vi "Excel_Open.vi"(8 "error in (no error)":errorcluster, 10 "template (empty)":path, 11 "excel application":refnum<k7>) -> (0 "error out":errorcluster, 3 "references":T1)   [LabVIEW 2015]
doc: "自己改的打开报表的工具"
panel:
  in  "Excel._Worksheet":refnum<k7>
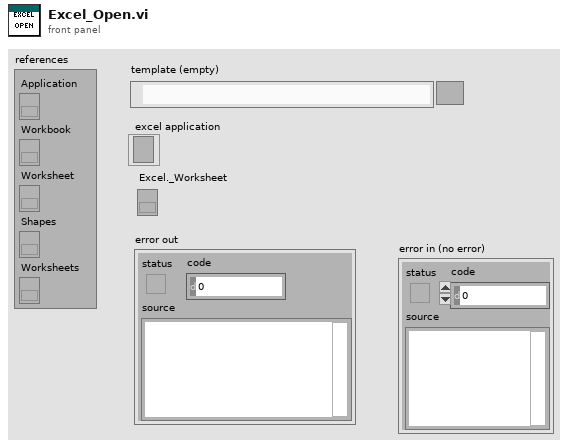
[diagram p1: front panel]
types:
  T1 = cluster{"Application":refnum<k7>, "Workbook":refnum<k7>, "Worksheet":refnum<k7>, "Shapes":refnum<k7>, "Worksheets":refnum<k7>}
  T2 = cluster{"excel application":refnum<k7>, "Add":refnum<k7>, "Excel._Worksheet":refnum<k7>, "Shapes":refnum<k7>, "Worksheets":refnum<k7>}
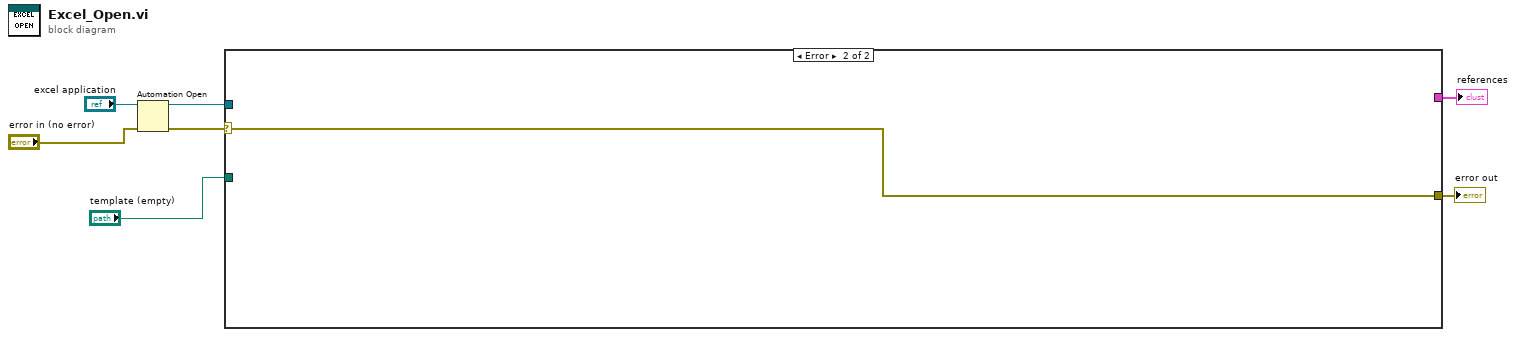
[diagram p0: block diagram]
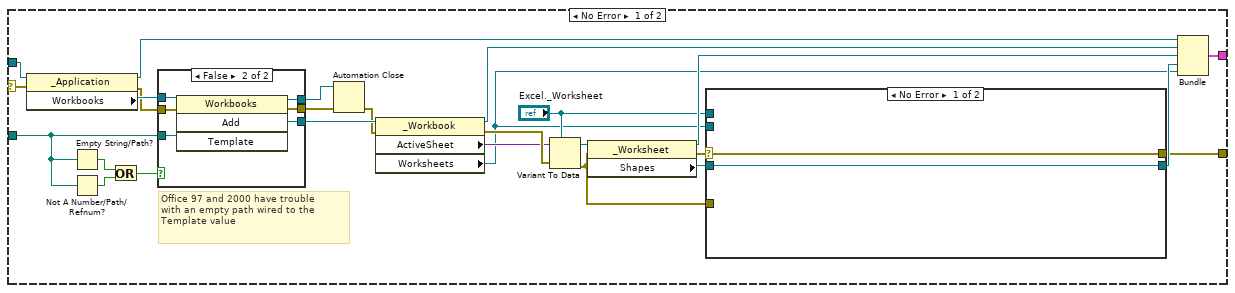
[diagram p2: hidden frame]
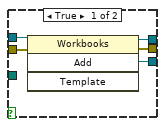
[diagram p3: hidden frame]
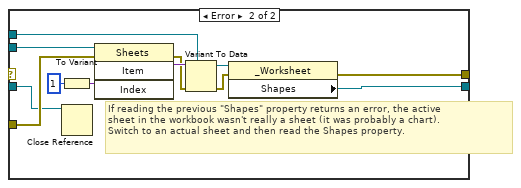
[diagram p4: hidden frame]
diagram:
  n1 = Automation Open(error in (no error)="error in (no error)", Automation Refnum="excel application") -> (Automation Refnum=w2:refnum<k7>, error out=w4:errorcluster)  [unwired: 2 in]
  n2 = case shown="Error" w4 {
    selector: w4 -> [w13 w59]
    tunnel: "template (empty)" -> [w12 _]
    tunnel: [w21 _] -> w6
    tunnel: [w16 w59] -> w3
    tunnel: w2 -> [w8 _]
    frame No Error {
      # "Office 97 and 2000 have trouble\nwith an empty path wired to the\nTemplate value"
      n3 = property class="_Application"(reference=w8, error in=w13) -> (reference out=w30:refnum<k7>, error out=w31:errorcluster, "Workbooks"=w32:refnum<k7>)
      n4 = Empty String/Path?(string/path=w12) -> (empty?=w11:bool)
      n5 = Not A Number/Path/Refnum?(number/path/refnum=w12) -> (NaN/Path/Refnum?=w10:bool)
      n6 = Or(x=w11, y=w10) -> (x .or. y?=w9:bool)
      n7 = case shown="False" w9 {
        tunnel: [w38 w44] -> w33
        tunnel: w32 -> [w37 w43]
        tunnel: w31 -> [w36 w42]
        tunnel: [w35 w41] -> w29
        tunnel: [w34 w40] -> w28
        tunnel: w12 -> [_ w39]
        frame True {
          n8 = invoke class="Workbooks" method="Add"(reference=w37, error in=w36) -> (reference out=w34:refnum<k7>, error out=w35:errorcluster, "Add"=w38:refnum<k7>)  [unwired: 2 in, 1 out]
        }
        frame False {
          n9 = invoke class="Workbooks" method="Add"(reference=w43, error in=w42, "Template"=w39) -> (reference out=w40:refnum<k7>, error out=w41:errorcluster, "Add"=w44:refnum<k7>)  [unwired: 1 in, 1 out]
        }
      }
      n10 = Automation Close(3:w29, 5:w28) -> (0:w27:errorcluster)
      n11 = property class="_Workbook"(reference=w33, error in=w27) -> (reference out=w23:refnum<k7>, error out=w26:errorcluster, "ActiveSheet"=w24:variant, "Worksheets"=w14:refnum<k7>)
      n12 = Variant To Data(error in=w26, type="Excel._Worksheet", Variant=w24) -> (data=w25:refnum<k7>, error out=w20:errorcluster)
      n13 = property class="_Worksheet"(reference=w25, error in=w20) -> (reference out=w22:refnum<k7>, error out=w17:errorcluster, "Shapes"=w19:refnum<k7>)
      n14 = case shown="No Error" w17 {
        selector: w17 -> [w46 _]
        tunnel: w14 -> [_ w55]
        tunnel: "Excel._Worksheet" -> [_ w53]
        tunnel: [w45 w52] -> w18
        tunnel: [w46 w51] -> w16
        tunnel: w20 -> [_ w50]
        tunnel: w19 -> [w45 w49]
        frame No Error {
        }
        frame Error {
          # "If reading the previous \"Shapes\" property returns an error, the active\nsheet in the workbook wasn't really a sheet (it was probably a chart).\nSwitch to an actual sheet and then read the Shapes property."
          n15 = To Variant(anything=1) -> (Variant=w57:variant)
          n16 = Close Reference(reference=w49) -> ()  [unwired: 1 in, 1 out]
          n17 = invoke class="Sheets" method="Item"(reference=w55, error in=w50, "Index"=w57) -> (error out=w54:errorcluster, "Item"=w58:variant)  [unwired: 1 in, 2 out]
          n18 = Variant To Data(error in=w54, type=w53, Variant=w58) -> (data=w48:refnum<k7>, error out=w47:errorcluster)
          n19 = property class="_Worksheet"(reference=w48, error in=w47) -> (error out=w51:errorcluster, "Shapes"=w52:refnum<k7>)  [unwired: 1 out]
        }
      }
      n20 = Bundle("excel application"=w30, "Add"=w23, "Excel._Worksheet"=w22, "Shapes"=w18, "Worksheets"=w14) -> (w21:T2)  [unwired: 1 out]
    }
    frame Error {
    }
  }
  "references" <- w6
  "error out" <- w3
